vi "Group Path.vi"(4 "Group Name":string) -> (7 "Group Path":path)   [LabVIEW 2020, in "User Prefs.lvlib" / "PrefsDB.lvclass"]
uses:
  PrefsDB.lvclass
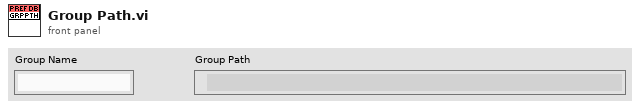
[diagram p1: front panel]
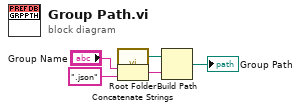
[diagram p0: block diagram]
diagram:
  n1 = call "Root Folder.vi"() -> ("Prefs Root"=w1:path)  [unwired: 7 in]
  n2 = Concatenate Strings("Group Name", ".json" ("string")) -> (w4:string)
  n3 = Build Path(base path=w1, name or relative path=w4) -> (appended path=→"Group Path":path)
